vi "Disconnect.vi"(8 "error in (no error)":errorcluster, 11 "BPC30x in":refnum<class "BPC30x.lvclass">) -> (0 "error out":errorcluster, 3 "BPC30x out":refnum<class "BPC30x.lvclass">)   [LabVIEW 2023, in "BPC30x.lvlib" / "BPC30x.lvclass"]
uses:
  BPC30x.lvclass
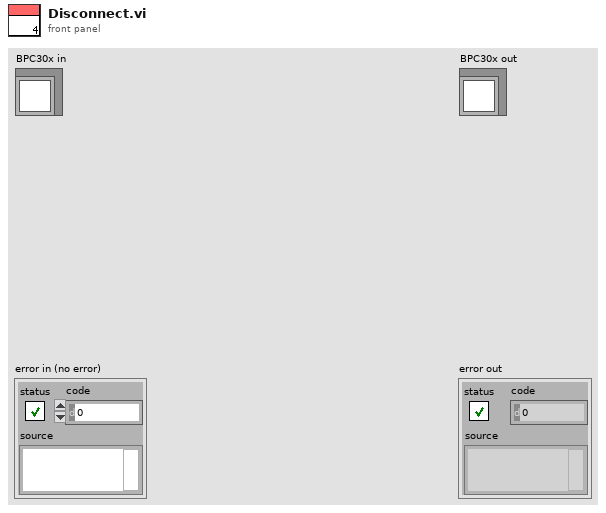
[diagram p1: front panel]
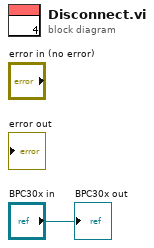
[diagram p0: block diagram]
diagram:
  "BPC30x out" <- "BPC30x in"
